vi "Dispose.vi"(8 "error in (no error)":errorcluster, 11 "IDispose":refnum<class "IDisposable.lvclass">) -> (0 "error out":errorcluster)   [LabVIEW 2020, in "IDisposable.lvclass"]
uses:
  IDisposable.lvclass
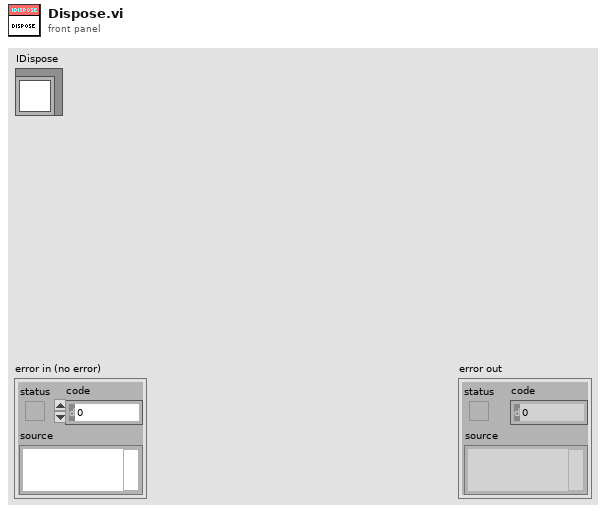
[diagram p1: front panel]
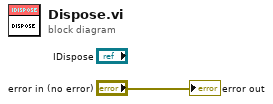
[diagram p0: block diagram]
diagram:
  "error out" <- "error in (no error)"
